vi "Create.vi"(8 "ErrorIn":errorcluster, 11 "ReferenceIn":refnum<class "TAFBaseGUI.lvclass">) -> (0 "ErrorOut":errorcluster, 3 "ReferenceOut":refnum<class "TAFBaseGUI.lvclass">)   [LabVIEW 2021, in "TAFBaseGUI.lvclass"]
doc: "Create the object instance"
uses:
  TAFBaseGUI.lvclass
  TAFBaseGUI.lvclass/TAFBaseGUI.ctl
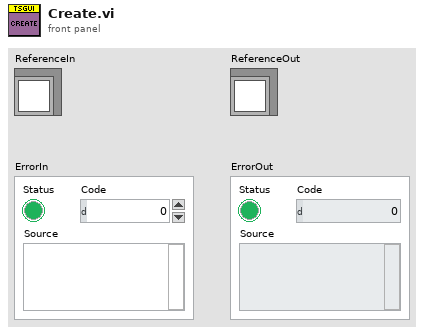
[diagram p1: front panel]
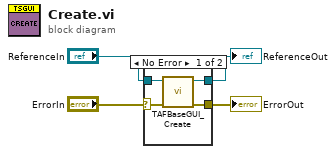
[diagram p0: block diagram]
diagram:
  n1 = case shown="No Error" "ErrorIn" {
    selector: "ErrorIn" -> [w8 w10]
    tunnel: [w7 w10] -> w3
    tunnel: [w5 w9] -> w1
    tunnel: "ReferenceIn" -> [w6 w9]
    frame No Error {
      n2 = call "TAFBaseGUI_Create.vi"("ErrorIn"=w8, "ReferenceIn"=w6) -> ("ErrorOut"=w7:errorcluster, "ReferenceOut"=w5:refnum<class "TAFBaseGUI.lvclass">)  [unwired: 8 in]
    }
    frame Error {
    }
  }
  "ErrorOut" <- w3
  "ReferenceOut" <- w1
